vi "Read VISA.vi"(8 "error in":errorcluster, 11 "VISA Refnum in":refnum<visa-resource-name>) -> (0 "error out":errorcluster, 1 "Display Time":picture, 2 "Command":string, 3 "VISA Refnum out":refnum<visa-resource-name>, 4 "File Save Time":string, 5 "Finish Connect?":bool, 7 "Start Connect?":bool)   [LabVIEW 2021]
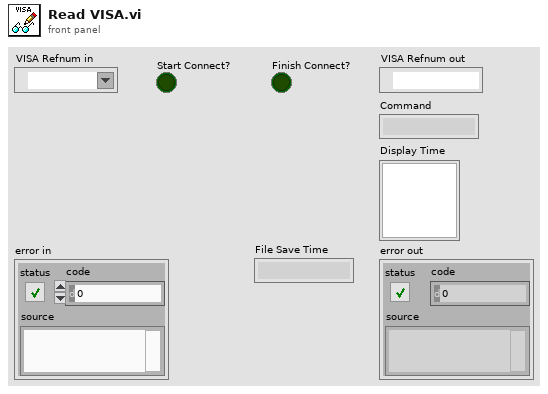
[diagram p1: front panel]
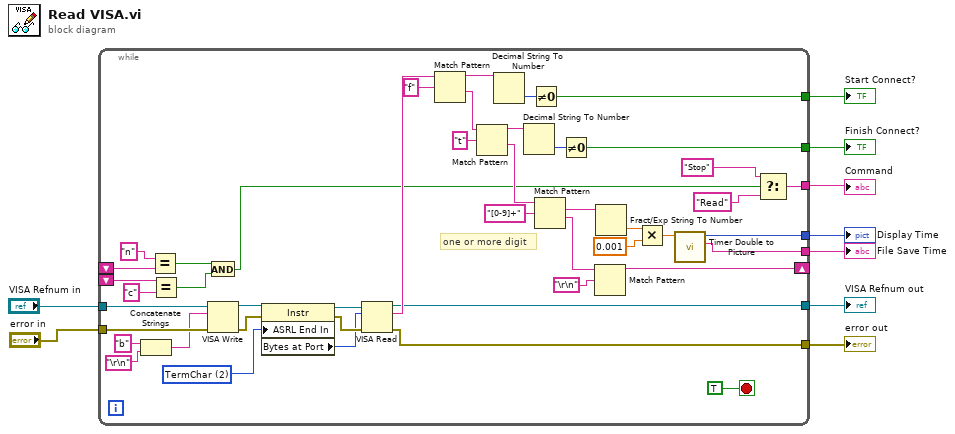
[diagram p0: block diagram]
diagram:
  n1 = while {
    tunnel: "VISA Refnum in" -> [w54]
    tunnel: "error in" -> [w53]
    tunnel: [w28] -> w7
    tunnel: [w27] -> w6
    tunnel: [w26] -> w5
    tunnel: [w25] -> w4
    shift-right: [w13] -> _
    shift-left: _ -> [w24]
    shift-left: _ -> [w22]
    tunnel: [w12] -> w3
    tunnel: [w11] -> w2
    tunnel: [w10] -> w1
    stop <- TRUE stop-if-true
    w37 = u16 2 items=["None", "Last Bit", "TermChar"] ("Serial Settings:End Mode for Reads")
    # "one or more digit"
    n2 = Concatenate Strings("b" ("write buffer"), "\r\n") -> (w52:string)
    n3 = Equal?(x="n", y=w24) -> (x = y?=w20:bool)
    n4 = Equal?(x=w22, y="c") -> (x = y?=w19:bool)
    n5 = And(x=w20, y=w19) -> (x .and. y?=w18:bool)
    n6 = VISA Write(VISA resource name=w54, write buffer=w52, error in (no error)=w53) -> (VISA resource name out=w41:refnum<visa-resource-name>, error out=w39:errorcluster)  [unwired: 1 out]
    n7 = property class="Instr"(reference=w41, error in=w39, "ASRL End In"=w37) -> (reference out=w40:refnum<visa-resource-name>, error out=w38:errorcluster, "Bytes at Port"=w36:u32)
    n8 = VISA Read(VISA resource name=w40, byte count=w36, error in (no error)=w38) -> (VISA resource name out=w26:refnum<visa-resource-name>, read buffer=w49:string, error out=w25:errorcluster)  [unwired: 1 out]
    n9 = Match Pattern(string=w49, regular expression="f") -> (before substring=w47:string, after substring=w44:string)  [unwired: 1 in, 2 out]
    n10 = Match Pattern(string=w44, regular expression="t") -> (before substring=w42:string, after substring=w31:string)  [unwired: 1 in, 2 out]
    n11 = Decimal String To Number(string=w47) -> (number=w46:i32)  [unwired: 2 in, 1 out]
    n12 = Decimal String To Number(string=w42) -> (number=w43:i32)  [unwired: 2 in, 1 out]
    n13 = Not Equal To 0?(x=w46) -> (x != 0?=w12:bool)
    n14 = Match Pattern(string=w31, regular expression="[0-9]+") -> (match substring=w30:string, after substring=w15:string)  [unwired: 1 in, 2 out]
    n15 = Not Equal To 0?(x=w43) -> (x != 0?=w11:bool)
    n16 = Match Pattern(string=w15, regular expression="\r\n") -> (before substring=w13:string)  [unwired: 1 in, 3 out]
    n17 = Fract/Exp String To Number(string=w30) -> (number=w33:dbl)  [unwired: 3 in, 1 out]
    n18 = Multiply(x=w33, y=0.001) -> (x*y=w34:dbl)
    n19 = call "Timer Double to Picture.vi"("Time (sec)"=w34) -> ("Time"=w10:string, "new picture"=w27:picture)  [unwired: 9 in]
    n20 = Select(t="Stop" ("regular expression"), s=w18, f="Read" ("regular expression")) -> (s? t:f=w28:string)
  }
  "Command" <- w7
  "error out" <- w4
  "VISA Refnum out" <- w5
  "Display Time" <- w6
  "Finish Connect?" <- w2
  "Start Connect?" <- w3
  "File Save Time" <- w1
